vi "RefIsOwner.vi"(10 "IsOwner?":refnum<vi>, 11 "MyRefsOwner":refnum<vi>) -> (1 "IsOwner?":bool, 2 "index":i32, 3 "Owner hierarchy (owner, grandowner)":refnum<vi>[](array[refnum]))   [LabVIEW 2019, in "BlueUtilityScripts.lvlib"]
uses:
  BlueUtilityScripts.lvlib
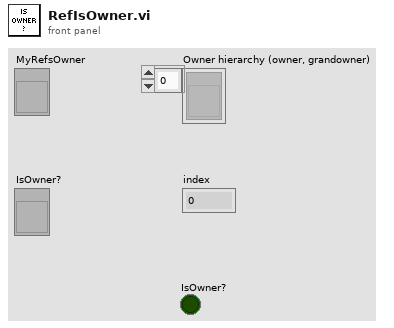
[diagram p1: front panel]
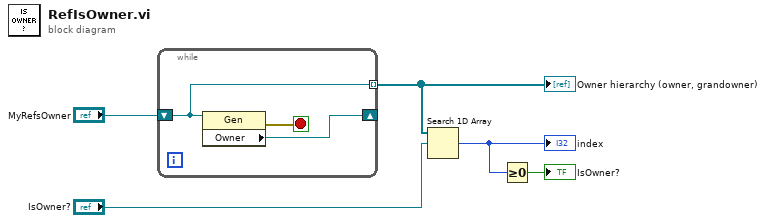
[diagram p0: block diagram]
diagram:
  n1 = while {
    shift-right: [w8] -> _
    shift-left: "MyRefsOwner" -> [w7]
    tunnel: [w7] -> w5 mode=indexing
    stop <- w6 stop-if-true
    n2 = property class="Gen"(reference=w7) -> (error out=w6:errorcluster, "Owner"=w8:refnum<vi>)  [unwired: 1 in, 1 out]
  }
  "Owner hierarchy (owner, grandowner)" <- w5
  n3 = Search 1D Array(1D array=w5, element="IsOwner?") -> (index of element=w2:i32)  [unwired: 1 in]
  "index" <- w2
  n4 = Greater Or Equal To 0?(x=w2) -> (x >= 0?=→"IsOwner?":bool)
